vi "Read U16.vi"(8 "error in":errorcluster, 10 "register name":string, 11 "session in":u32) -> (0 "error out":errorcluster, 2 "value out":u16, 3 "session out":u32)   [LabVIEW 2018, in "Scalar IO Operations.lvlib"]
uses:
  Scalar IO Operations.lvlib
  NiFpga.dll
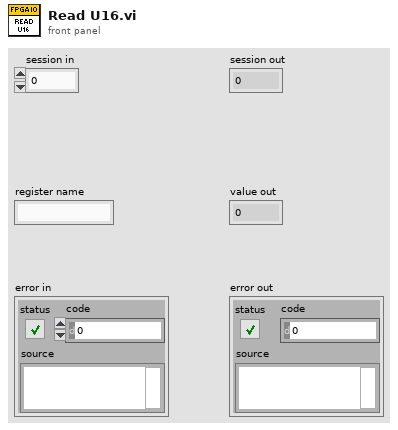
[diagram p1: front panel]
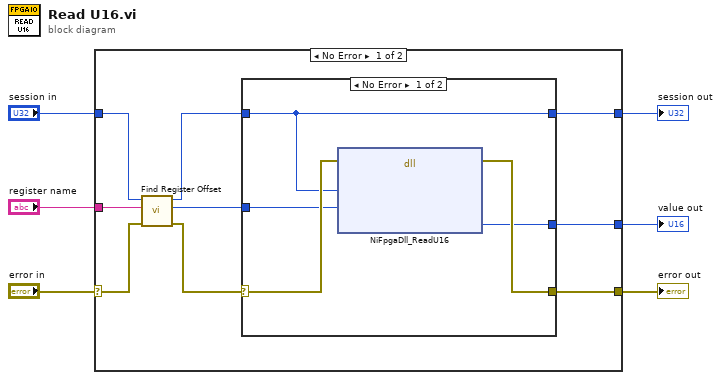
[diagram p0: block diagram]
diagram:
  n1 = case shown="No Error" "error in" {
    selector: "error in" -> [w7 w23]
    tunnel: [w15 w24] -> w6
    tunnel: [w14 w23] -> w5
    tunnel: [w13 _] -> w4
    tunnel: "session in" -> [w10 w24]
    tunnel: "register name" -> [w8 _]
    frame No Error {
      n2 = call "Find Register Offset.vi"("error in (no error)"=w7, "register name"=w8, "session in"=w10) -> ("error out"=w11:errorcluster, "resource offset"=w12:u32, "session out"=w9:u32)  [unwired: 6 in]
      n3 = case shown="No Error" w11 {
        selector: w11 -> [w20 w22]
        tunnel: w9 -> [w19 w21]
        tunnel: [w17 w22] -> w14
        tunnel: [w16 _] -> w13
        tunnel: w12 -> [w18 _]
        tunnel: [w19 w21] -> w15
        frame No Error {
          n4 = dll-call lib="NiFpga.*" fn="NiFpgaDll_ReadU16"(error in=w20, "session"=w19, "offset"=w18) -> (error out=w17:errorcluster, "value"=w16:u16)  [unwired: 6 in, 1 out]
        }
        frame Error {
        }
      }
    }
    frame Error {
    }
  }
  "error out" <- w5
  "session out" <- w6
  "value out" <- w4
